vi "modify.vi"(8 "error in (no error)":errorcluster, 11 "GenericTrajectory in":refnum<class "GenericTrajectory.lvclass">) -> (0 "error out":errorcluster, 3 "GenericTrajectory out":refnum<class "GenericTrajectory.lvclass">)   [LabVIEW 2010, in "GenericTrajectory.lvclass"]
uses:
  GenericTrajectory.lvclass
panel:
  # "This functionality is not implemented for your configuration."
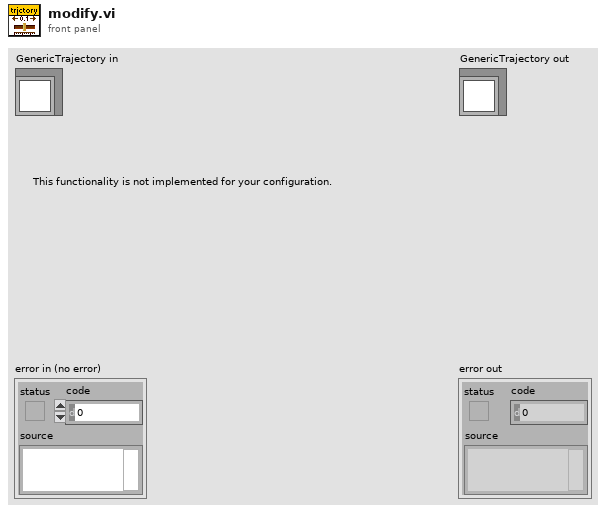
[diagram p1: front panel]
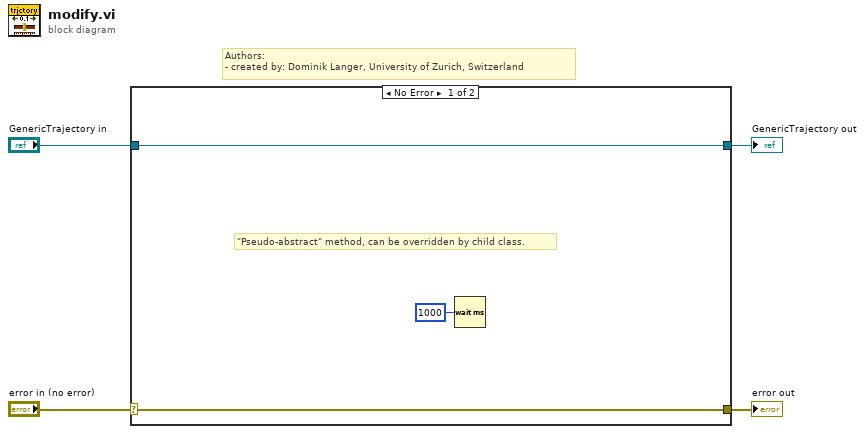
[diagram p0: block diagram]
diagram:
  # "Authors: \n- created by: Dominik Langer, University of Zurich, Switzerland"
  n1 = case shown="No Error" "error in (no error)" {
    selector: "error in (no error)" -> [w6 w9]
    tunnel: [w6 w9] -> w3
    tunnel: [w7 w8] -> w1
    tunnel: "GenericTrajectory in" -> [w7 w8]
    frame No Error {
      # "\"Pseudo-abstract\" method, can be overridden by child class."
      n2 = Wait (ms)(milliseconds to wait=u32 1000) -> ()  [unwired: 1 out]
    }
    frame Error {
    }
  }
  "error out" <- w3
  "GenericTrajectory out" <- w1
